vi "Deplacement avance-recule.vi"() -> ()   [LabVIEW 2019]
uses:
  <vilib>/Rock Robotics/WPI/ThirdParty/Phoenix-LabVIEW/Motor Controller/Get/CTRE_Phoenix_MotorController_GetQuadratureData.vi
  <vilib>/addons/control/pid/pid.llb/PID (DBL).vi
  Global.vi
  <vilib>/addons/control/pid/NI_PID_pid.lvlib
panel:
  in  "Deplacement (m)":dbl
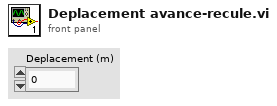
[diagram p1: front panel]
types:
  T1 = cluster{"proportional gain (Kc)":dbl, "integral time (Ti, min)":dbl, "derivative time (Td, min)":dbl}
  T2 = typedef "WPI_MotorControlDeviceRef.ctl" = cluster{"DeviceStatus":errorcluster, "Type":T3, "PWM":cluster{"PWM Channel":T4, "DeadBand":T5}, "CAN":cluster{"Device Number":u8, "SetOutput VI Ref":variant, "GetOutput VI Ref":variant, "Enable VI Ref":variant, "Disable VI Ref":variant, "Data":variant}, "Invert":bool, "DIO PWM":cluster{"PWM \"Enable\" Channel":T4, "DIOChannel":T6, "PWM Rate":dbl}}
  T3 = typedef "WPI_MotorControlType.ctl" = enum16{"PWM", "CAN", "DIO PWM"}
  T4 = typedef "FPGA_DIOPWMChannel.ctl" = enum8{"PWM 0", "PWM 1", "PWM 2", "PWM 3", "PWM 4", "PWM 5", "PWM 6", "PWM 7", "PWM 8", "PWM 9", "PWM MXP 0", "PWM MXP 1", "PWM MXP 2", "PWM MXP 3", "PWM MXP 4", "PWM MXP 5", "PWM MXP 6", "PWM MXP 7", "PWM MXP 8", "PWM MXP 9", "Invalid"}
  T5 = typedef "WPI_PWMDeadband.ctl" = cluster{"Name":string, "maxPositivePwm":i32, "minPositivePwm":i32, "centerPwm":i32, "maxNegativePwm":i32, "minNegativePwm":i32, "angularRange":u16}
  T6 = typedef "FPGA_DIOChannel.ctl" = enum8{"DIO 0", "DIO 1", "DIO 2", "DIO 3", "DIO 4", "DIO 5", "DIO 6", "DIO 7", "DIO 8", "DIO 9", "DIO MXP 0", "DIO MXP 1", "DIO MXP 2", "DIO MXP 3", "DIO MXP 4", "DIO MXP 5", "DIO MXP 6", "DIO MXP 7", "DIO MXP 8", "DIO MXP 9", "DIO MXP 10", "DIO MXP 11", "DIO MXP 12", "DIO MXP 13", "DIO MXP 14", "DIO MXP 15", "SPI Port CS1", "SPI Port CS2", "SPI Port CS3", "SPI Port MISO", "SPI Port MOSI", "Invalid"}
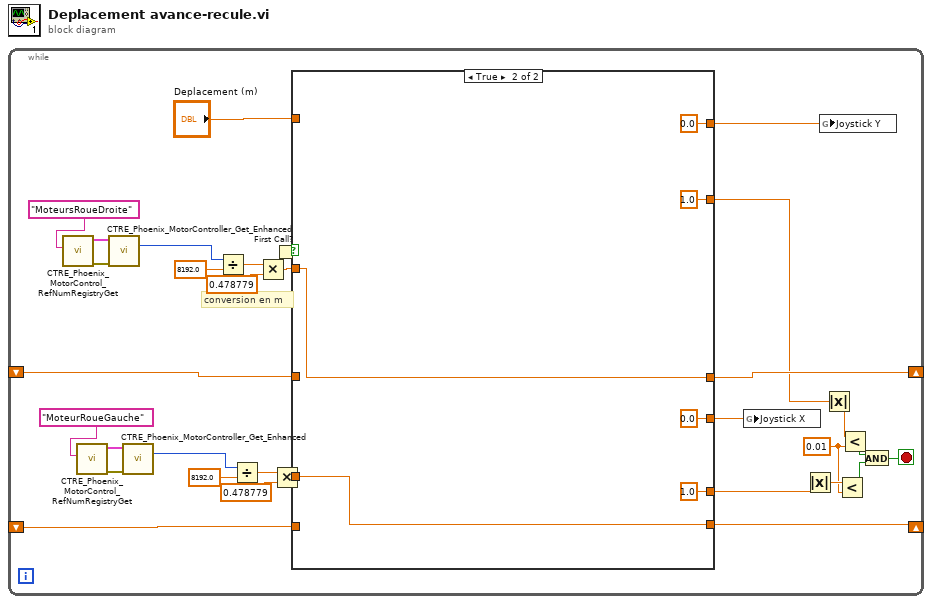
[diagram p0: block diagram]
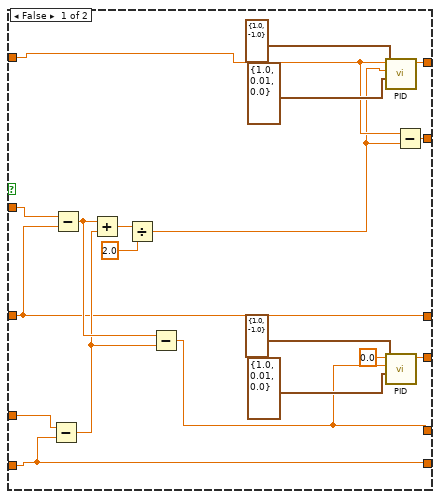
[diagram p2: hidden frame]
diagram:
  n1 = while {
    shift-right: [w31] -> _
    shift-left: _ -> [w30]
    shift-right: [w9] -> _
    shift-left: _ -> [w8]
    stop <- w5 stop-if-true
    w2 = 0.01 ("y")
    # "conversion en m"
    n2 = call <vilib>:"CTRE_Phoenix_MotorControl_RefNumRegistryGet.vi"("refnum name"="MoteursRoueDroite") -> ("error out"=w20:errorcluster, "PhoenixMotorControlDevRef"=w19:T2)  [unwired: 9 in]
    n3 = call <vilib>:"CTRE_Phoenix_MotorControl_RefNumRegistryGet.vi"("refnum name"="MoteurRoueGauche") -> ("error out"=w13:errorcluster, "PhoenixMotorControlDevRef"=w12:T2)  [unwired: 9 in]
    n4 = call-poly <vilib>:"CTRE_Phoenix_MotorController_Get_Enhanced.vi"("PhoenixMotorControlDevRef"=w19, "error in"=w20) -> ("Quadrature Position"=w21:i32)  [unwired: 10 in, 3 out]
    n5 = call-poly <vilib>:"CTRE_Phoenix_MotorController_Get_Enhanced.vi"("PhoenixMotorControlDevRef"=w12, "error in"=w13) -> ("Quadrature Position"=w14:i32)  [unwired: 10 in, 3 out]
    n6 = Divide(x=w21, y=8192.0) -> (x/y=w25:dbl)
    n7 = Divide(x=w14, y=8192.0) -> (x/y=w17:dbl)
    n8 = Multiply(x=w25, y=0.478779) -> (x*y=w23:dbl)
    n9 = First Call?() -> (First Call?: T/F=w32:bool)
    n10 = Multiply(x=w17, y=0.478779) -> (x*y=w10:dbl)
    n11 = case shown="True" w32 {
      tunnel: w23 -> [w46 w55]
      tunnel: [w39 w55] -> w31
      tunnel: w30 -> [w39 _]
      tunnel: "Deplacement (m)" -> [w48 _]
      tunnel: [w49 0.0 ("output")] -> w28
      tunnel: [w47 1.0] -> w27
      tunnel: w10 -> [w45 w54]
      tunnel: [w38 w54] -> w9
      tunnel: w8 -> [w38 _]
      tunnel: [w34 1.0] -> w7
      tunnel: [w33 0.0 ("output")] -> w1
      frame False {
        n12 = Subtract(x=w45, y=w38) -> (x-y=w40:dbl)
        n13 = Subtract(x=w46, y=w39) -> (x-y=w41:dbl)
        n14 = Add(x=w41, y=w40) -> (x+y=w44:dbl)
        n15 = Divide(x=w44, y=2.0) -> (x/y=w42:dbl)
        n16 = Subtract(x=w41, y=w40) -> (x-y=w34:dbl)
        n17 = call-poly <vilib>:"PID.vi"("output range"=cluster{"output high":dbl, "output low":dbl} {"output high"=1.0, "output low"=-1.0}, "PID gains"=T1 {"proportional gain (Kc)"=1.0, "integral time (Ti, min)"=0.01, "derivative time (Td, min)"=0.0}, "process variable"=w42, "setpoint"=w48) -> ("output"=w49:dbl)  [unwired: 6 in, 1 out]
        n18 = call-poly <vilib>:"PID.vi"("output range"=cluster{"output high":dbl, "output low":dbl} {"output high"=1.0, "output low"=-1.0}, "PID gains"=T1 {"proportional gain (Kc)"=1.0, "integral time (Ti, min)"=0.01, "derivative time (Td, min)"=0.0}, "process variable"=w34, "setpoint"=0.0) -> ("output"=w33:dbl)  [unwired: 6 in, 1 out]
        n19 = Subtract(x=w48, y=w42) -> (x-y=w47:dbl)
      }
      frame True {
      }
    }
    n20 = global write "Global.vi" "Joystick X"(w1) -> ()
    n21 = Absolute Value(x=w7) -> (abs(x)=w6:dbl)
    n22 = global write "Global.vi" "Joystick Y"(w28) -> ()
    n23 = Absolute Value(x=w27) -> (abs(x)=w26:dbl)
    n24 = Less?(x=w6, y=w2) -> (x < y?=w3:bool)
    n25 = Less?(x=w26, y=w2) -> (x < y?=w4:bool)
    n26 = And(x=w4, y=w3) -> (x .and. y?=w5:bool)
  }
